vi "Configuration0.vi"() -> ()   [LabVIEW 2016]
uses:
  <vilib>/MakerHub/LINX/Public/Peripherals/Digital/Digital Write 1 Chan.vi
  <vilib>/MakerHub/LINX/Public/Peripherals/Digital/Digital Write N Chans.vi
  <vilib>/MakerHub/LINX/Private/Local IO/LinxDigitalWrite.vi
  <vilib>/MakerHub/LINX/Public/Utilities/Check Channel.vi
  <vilib>/MakerHub/LINX/Public/Utilities/Open Serial.vi
  <vilib>/MakerHub/LINX/Private/Utilties/Generate Error.vi
  <vilib>/MakerHub/LINX/LMH-LINX.lvlib
panel:
  in  "Pin#":u8=46
  in  "Pin#":u8=42
  in  "Pin#":u8=41
  in  "Pin#":u8=36
  in  "Pin#":u8=35
  in  "Pin#":u8=40
  in  "Pin#":u8=34
  in  "Pin#":u8=45
  in  "Pin#":u8=44
  in  "Pin#":u8=43
  in  "Pin#":u8=39
  in  "Pin#":u8=33
  in  "Pin#":u8=38
  in  "Pin#":u8=37
  in  "Pin#":u8=32
  in  "Pin#":u8=31
  in  "Arduino Port":refnum<visa-resource-name>="COM5"
  # "Set Relay Pins (then set to default under EDIT)"
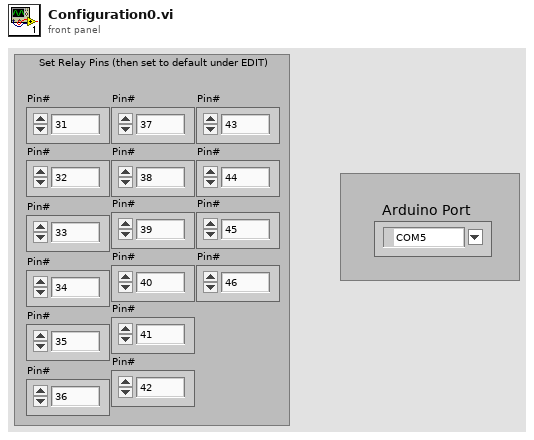
[diagram p1: front panel]
types:
  T1 = typedef "LMH-LINX.lvlib/LINX Ref.ctl" = cluster{"IO":T2, "Interface":T3, "LINX Device Config":T4}
  T2 = typedef "LMH-LINX.lvlib/Platform.ctl" = enum16{"Remote", "Local"}
  T3 = typedef "LMH-LINX.lvlib/Interface.ctl" = enum16{"Serial", "TCP"}
  T4 = typedef "LMH-LINX.lvlib/Device.lvlib/LINX Device Config.ctl" = cluster{"Interface":T3, "COM Port":refnum<visa-resource-name>, "TCP Configuration":T5, "Device Family":u8, "Device ID":u8, "Device Name":string, "TCP Ref":refnum<k5>, "Channels":T6}
  T5 = typedef "LMH-LINX.lvlib/Device.lvlib/TCP Config.ctl" = cluster{"IP Address":string, "Port":u16}
  T6 = typedef "LMH-LINX.lvlib/Channels.ctl" = cluster{"DI":u8[], "DO":u8[], "AI":u8[], "AO":u8[], "PWM":u8[], "QE":u8[], "UART":u8[], "I2C 2":u8[], "SPI":u8[], "CAN":u8[], "Servo":u8[], "AI Ref (V)":dbl, "AI Resolution (Bits)":u8, "AO Ref (V)":dbl, "AO Resolution (Bits)":u8}
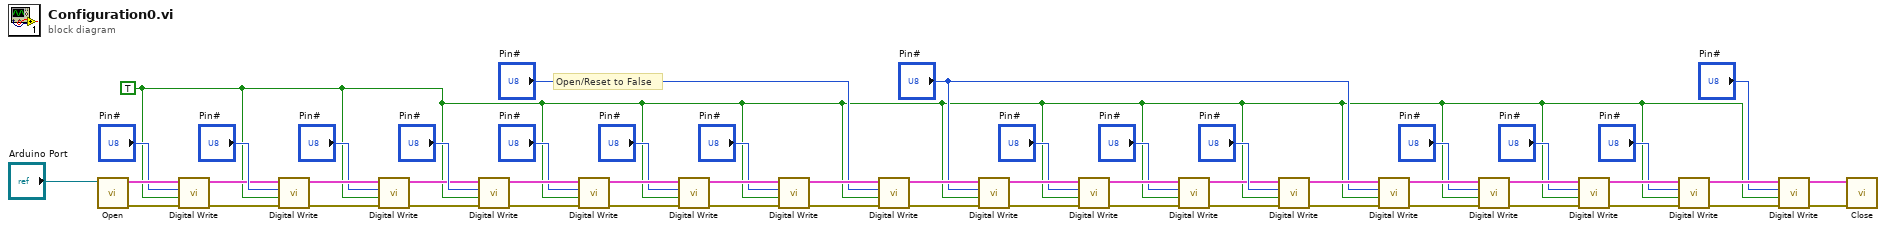
[diagram p0: block diagram]
diagram:
  w4 = TRUE
  # "Open/Reset to False"
  n1 = call-poly <vilib>:"Open.vi"("Serial Port"="Arduino Port") -> ("Error Out"=w52:errorcluster, "LINX Resource"=w53:T1)  [unwired: 8 in, 1 out]
  n2 = call-poly <vilib>:"Digital Write.vi"("Error In"=w52, "Output Value"=w4, "DO Channel"="Pin#", "LINX Resource"=w53) -> ("Error Out"=w48:errorcluster, "LINX Resource"=w49:T1)  [unwired: 6 in]
  n3 = call-poly <vilib>:"Digital Write.vi"("Error In"=w48, "Output Value"=w4, "DO Channel"="Pin#", "LINX Resource"=w49) -> ("Error Out"=w46:errorcluster, "LINX Resource"=w47:T1)  [unwired: 6 in]
  n4 = call-poly <vilib>:"Digital Write.vi"("Error In"=w46, "Output Value"=w4, "DO Channel"="Pin#", "LINX Resource"=w47) -> ("Error Out"=w42:errorcluster, "LINX Resource"=w43:T1)  [unwired: 6 in]
  n5 = call-poly <vilib>:"Digital Write.vi"("Error In"=w42, "Output Value"=w4, "DO Channel"="Pin#", "LINX Resource"=w43) -> ("Error Out"=w40:errorcluster, "LINX Resource"=w41:T1)  [unwired: 6 in]
  n6 = call-poly <vilib>:"Digital Write.vi"("Error In"=w40, "Output Value"=w4, "DO Channel"="Pin#", "LINX Resource"=w41) -> ("Error Out"=w37:errorcluster, "LINX Resource"=w38:T1)  [unwired: 6 in]
  n7 = call-poly <vilib>:"Digital Write.vi"("Error In"=w37, "Output Value"=w4, "DO Channel"="Pin#", "LINX Resource"=w38) -> ("Error Out"=w34:errorcluster, "LINX Resource"=w35:T1)  [unwired: 6 in]
  n8 = call-poly <vilib>:"Digital Write.vi"("Error In"=w34, "Output Value"=w4, "DO Channel"="Pin#", "LINX Resource"=w35) -> ("Error Out"=w31:errorcluster, "LINX Resource"=w32:T1)  [unwired: 6 in]
  n9 = call-poly <vilib>:"Digital Write.vi"("Error In"=w31, "Output Value"=w4, "DO Channel"="Pin#", "LINX Resource"=w32) -> ("Error Out"=w28:errorcluster, "LINX Resource"=w29:T1)  [unwired: 6 in]
  n10 = call-poly <vilib>:"Digital Write.vi"("Error In"=w28, "Output Value"=w4, "DO Channel"="Pin#", "LINX Resource"=w29) -> ("Error Out"=w26:errorcluster, "LINX Resource"=w27:T1)  [unwired: 6 in]
  n11 = call-poly <vilib>:"Digital Write.vi"("Error In"=w26, "Output Value"=w4, "DO Channel"="Pin#", "LINX Resource"=w27) -> ("Error Out"=w23:errorcluster, "LINX Resource"=w24:T1)  [unwired: 6 in]
  n12 = call-poly <vilib>:"Digital Write.vi"("Error In"=w23, "Output Value"=w4, "DO Channel"="Pin#", "LINX Resource"=w24) -> ("Error Out"=w20:errorcluster, "LINX Resource"=w19:T1)  [unwired: 6 in]
  n13 = call-poly <vilib>:"Digital Write.vi"("Error In"=w20, "Output Value"=w4, "DO Channel"="Pin#", "LINX Resource"=w19) -> ("Error Out"=w17:errorcluster, "LINX Resource"=w18:T1)  [unwired: 6 in]
  n14 = call-poly <vilib>:"Digital Write.vi"("Error In"=w17, "Output Value"=w4, "DO Channel"="Pin#", "LINX Resource"=w18) -> ("Error Out"=w14:errorcluster, "LINX Resource"=w15:T1)  [unwired: 6 in]
  n15 = call-poly <vilib>:"Digital Write.vi"("Error In"=w14, "Output Value"=w4, "DO Channel"="Pin#", "LINX Resource"=w15) -> ("Error Out"=w11:errorcluster, "LINX Resource"=w12:T1)  [unwired: 6 in]
  n16 = call-poly <vilib>:"Digital Write.vi"("Error In"=w11, "Output Value"=w4, "DO Channel"="Pin#", "LINX Resource"=w12) -> ("Error Out"=w8:errorcluster, "LINX Resource"=w9:T1)  [unwired: 6 in]
  n17 = call-poly <vilib>:"Digital Write.vi"("Error In"=w8, "Output Value"=w4, "DO Channel"="Pin#", "LINX Resource"=w9) -> ("Error Out"=w3:errorcluster, "LINX Resource"=w6:T1)  [unwired: 6 in]
  n18 = call-poly <vilib>:"Digital Write.vi"("Error In"=w3, "Output Value"=w4, "DO Channel"="Pin#", "LINX Resource"=w6) -> ("Error Out"=w1:errorcluster, "LINX Resource"=w2:T1)  [unwired: 6 in]
  n19 = call <vilib>:"Close.vi"("Error In"=w1, "LINX Resource"=w2) -> ()  [unwired: 9 in, 1 out]
